vi "Write to Port.vi"(8 "error in":errorcluster, 10 "Data":string) -> (0 "error out":errorcluster, 3 "Response Queue":refnum<queue>)   [LabVIEW 2019, in "Binary Actor.lvlib"]
uses:
  Binary Actor.lvlib
  Actor Task.ctl
  Actor Command.ctl
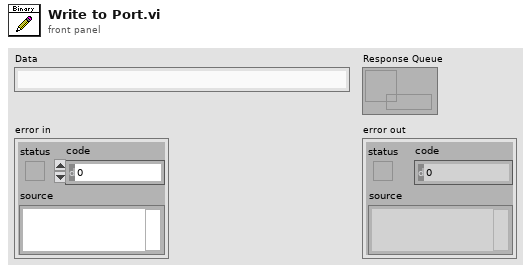
[diagram p1: front panel]
types:
  T1 = typedef "Binary Actor.lvlib/Actor Task.ctl" = enum8{"Write", "Get Data", "Stop"}
  T2 = typedef "Binary Actor.lvlib/Actor Command.ctl" = cluster{"Task":T1, "Data":string, "Response Queue":refnum<queue>}
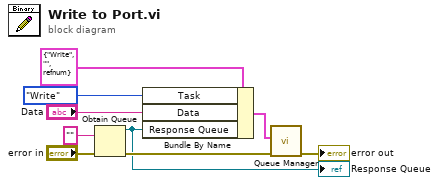
[diagram p0: block diagram]
diagram:
  n1 = Obtain Queue(element data type="", error in (no error)="error in") -> (queue out=w1:refnum<queue>, error out=w7:errorcluster)  [unwired: 3 in, 1 out]
  "Response Queue" <- w1
  n2 = Bundle By Name(cluster=T2 {"Task"=enum."Write", "Data"="", "Response Queue"=refnum} ("Command"), "Task"=Actor_Task."Write", "Data"="Data", "Response Queue"=w1) -> (w3:T2)
  n3 = call "Queue Manager.vi"("error in"=w7, "Command"=w3) -> ("error out"=→"error out":errorcluster)  [unwired: 8 in, 1 out]
